vi "nonfinite_constants.vi"() -> (1 "negative_inf":dbl=-inf, 2 "positive_inf":dbl=inf, 3 "nan_result":dbl=nan)   [LabVIEW 2020]
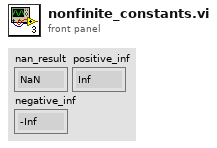
[diagram p1: front panel]
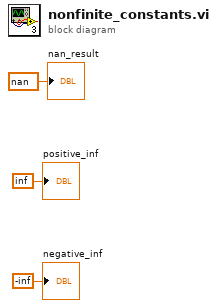
[diagram p0: block diagram]
diagram:
  "nan_result" <- nan
  "positive_inf" <- inf
  "negative_inf" <- -inf
